vi "Write Servo Channel.vi"(8 "error in (no error)":errorcluster, 10 "servo phys chan":tag, 11 "DAQmx Servo in":refnum<class "DAQmx Servo.lvclass">) -> (0 "error out":errorcluster, 3 "DAQmx Servo out":refnum<class "DAQmx Servo.lvclass">)   [LabVIEW 2020, in "DAQmx Servo.lvclass"]
uses:
  DAQmx Servo.lvclass
  DAQmx Servo.lvclass/DAQmx Servo.ctl
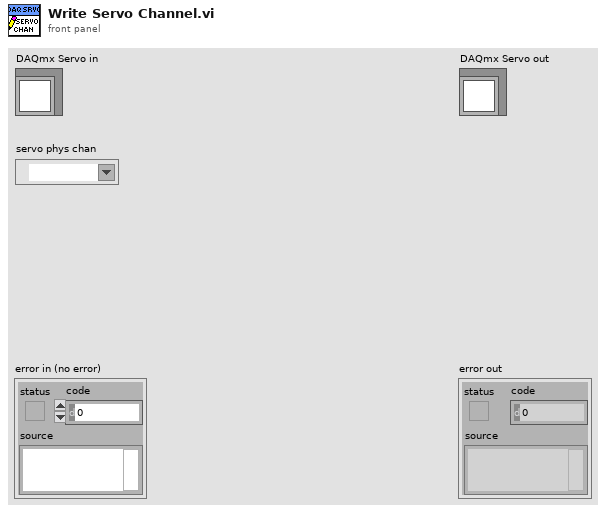
[diagram p1: front panel]
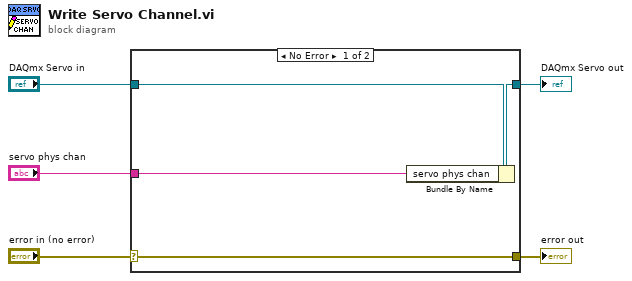
[diagram p0: block diagram]
diagram:
  n1 = case shown="No Error" "error in (no error)" {
    selector: "error in (no error)" -> [w9 w10]
    tunnel: [w9 w10] -> w4
    tunnel: [w7 w11] -> w2
    tunnel: "DAQmx Servo in" -> [w8 w11]
    tunnel: "servo phys chan" -> [w6 _]
    frame No Error {
      n2 = Bundle By Name(cluster=w8, "servo phys chan"=w6) -> (w7:refnum<class "DAQmx Servo.lvclass">)
    }
    frame Error {
    }
  }
  "error out" <- w4
  "DAQmx Servo out" <- w2
